vi "Table-Prevent out of range changes.vi"(8 "error in (no error)":errorcluster, 10 "Table Value in":string[][](array[string]), 11 "Table ref in":refnum<vi>) -> (0 "error out":errorcluster, 2 "Table Value out":string[][](array[string]), 3 "Table ref out":refnum<vi>)   [LabVIEW 2013]
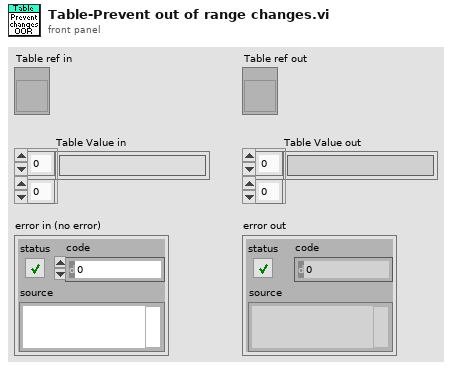
[diagram p1: front panel]
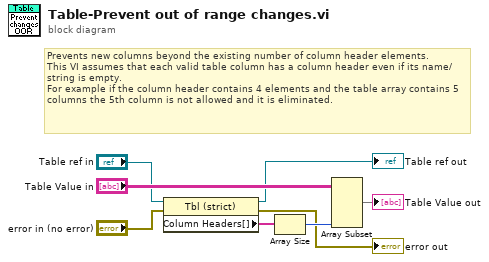
[diagram p0: block diagram]
diagram:
  # "Prevents new columns beyond the existing number of column header elements.\nThis VI assumes that each valid table column has a column header even if its name/string is empty.\nFor example if the column header contains 4 elements and the table array contains 5 columns the 5th column is not allowed and it is eliminated."
  n1 = property on="Property Node" class="Tbl (strict)"(reference="Table ref in", error in="error in (no error)") -> (reference out=→"Table ref out":refnum<vi>, error out=→"error out":errorcluster, "Column Headers[]"=w8:string[])
  n2 = Array Size(array=w8) -> (size(s)=w6:i32)
  n3 = Array Subset(array="Table Value in", length (col)=w6) -> (→"Table Value out":string[][])  [unwired: 3 in]
